vi "Recibir.vi"() -> ()   [LabVIEW 2020]
uses:
  <vilib>/httpClient/LabVIEWHTTPClient.lvlib
panel:
  out "Led Rele":bool
  out "hora 2":string
  out "hora":string
  out "Data":string
  out "Feedback (mA)":dbl
  in  "stop":bool
  out "error GET":errorcluster
  out "headers GET":string
  out "body GET":string
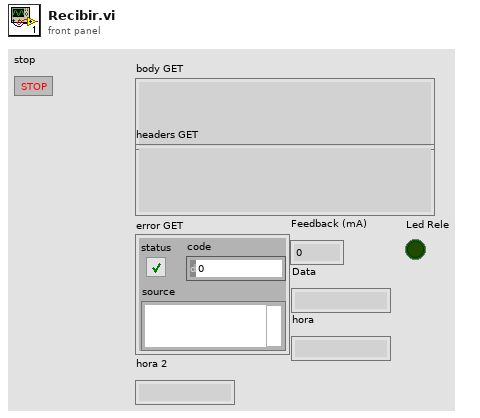
[diagram p1: front panel]
types:
  T1 = cluster{"Acionamiento":dbl, "Data":string, "Hora":string, "Rele":bool}
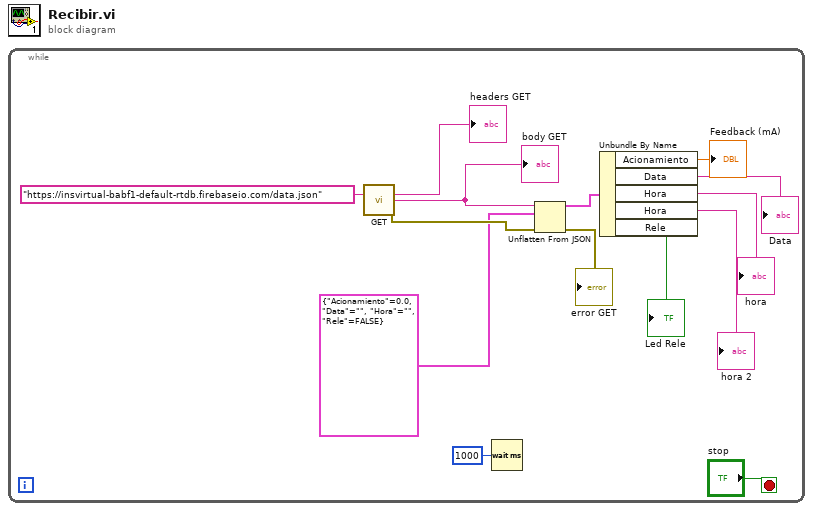
[diagram p0: block diagram]
diagram:
  n1 = while {
    stop <- "stop" stop-if-true
    n2 = call <vilib>:"GET.vi"("url"="https://insvirtual-babf1-default-rtdb.firebaseio.com/data.json") -> ("headers"=→"headers GET":string, "body"=w11:string, "error out"=w13:errorcluster)  [unwired: 11 in, 1 out]
    "body GET" <- w11
    n3 = Wait (ms)(milliseconds to wait=u32 1000) -> ()  [unwired: 1 out]
    n4 = Unflatten From JSON(JSON string=w11, type and defaults=T1 {"Acionamiento"=0.0, "Data"="", "Hora"="", "Rele"=FALSE}, error in (no error)=w13) -> (value=w6:T1, error out=→"error GET":errorcluster)  [unwired: 4 in]
    n5 = Unbundle By Name(w6) -> ("Acionamiento"=→"Feedback (mA)":dbl, "Data"=→"Data":string, "Hora"=→"hora":string, "Hora"=→"hora 2":string, "Rele"=→"Led Rele":bool)
  }
